vi "user initialization.vi"(8 "error in":errorcluster, 10 "configuration in":refnum<class "control module configuration.lvclass">, 11 "fixed channel runtime in":refnum<class "fixed channel runtime.lvclass">) -> (0 "error out":errorcluster, 3 "fixed channel runtime out":refnum<class "fixed channel runtime.lvclass">)   [LabVIEW 2013, in "fixed channel runtime.lvclass"]
uses:
  fixed channel runtime.lvclass
  <vilib>/NI/DCAF/Tag Editor Core/control module/configuration/control module configuration.lvclass
  configuration/fixed channel configuration.lvclass
  <vilib>/NI/DCAF/Tag Editor Core/control module/runtime/control module runtime.lvclass
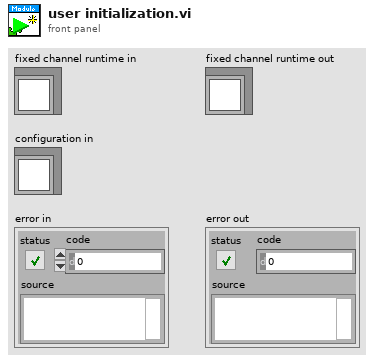
[diagram p1: front panel]
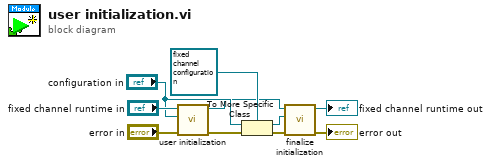
[diagram p0: block diagram]
diagram:
  n1 = call-parent "user initialization.vi"("error in"="error in", "configuration in"="configuration in", "fixed channel runtime in"="fixed channel runtime in") -> ("error out"=w8:errorcluster, "fixed channel runtime out"=w4:refnum<class "fixed channel runtime.lvclass">)  [unwired: 7 in]
  n2 = To More Specific Class(target class=refnum<class "fixed channel configuration.lvclass"> refnum ("fixed channel configuration"), reference="configuration in", error in=w8) -> (specific class reference=w3:refnum<class "fixed channel configuration.lvclass">, error out=w6:errorcluster)
  n3 = call-dynamic "finalize initialization.vi"("error in"=w6, "configuration in"=w3, "fixed channel runtime in"=w4) -> ("error out"=→"error out":errorcluster, "fixed channel runtime out"=→"fixed channel runtime out":refnum<class "fixed channel runtime.lvclass">)  [unwired: 7 in]
